vi "MFCCMD.vi"(8 "error in (no error)":errorcluster, 9 "cmd":string, 10 "Device ID's":string[](array[string]), 11 "VISA Refnum in":refnum<visa-resource-name>) -> (0 "error out":errorcluster, 3 "VISA Refnum out":refnum<visa-resource-name>)   [LabVIEW 2020, in "MFC.lvclass"]
uses:
  MFC/MFC.lvclass
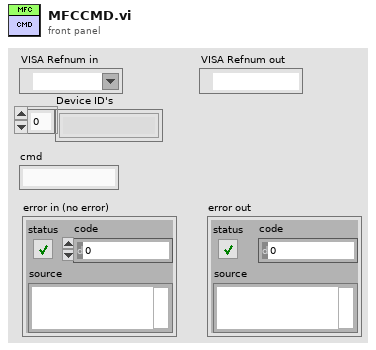
[diagram p1: front panel]
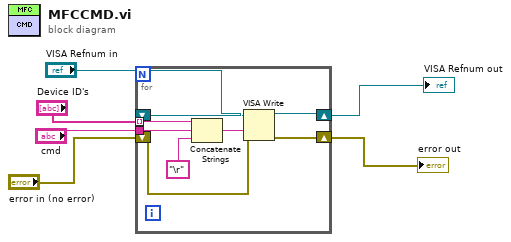
[diagram p0: block diagram]
diagram:
  n1 = for {
    tunnel: "Device ID's" -> [w12] mode=indexing
    shift-right: [w7] -> w5
    shift-left: "error in (no error)" -> [w14]
    shift-right: [w8] -> w6
    shift-left: "VISA Refnum in" -> [w13]
    tunnel: "cmd" -> [w10]
    n2 = Concatenate Strings(w12, w10, "\r" ("string")) -> (w11:string)
    n3 = VISA Write(VISA resource name=w13, write buffer=w11, error in (no error)=w14) -> (VISA resource name out=w8:refnum<visa-resource-name>, error out=w7:errorcluster)  [unwired: 1 out]
  }
  "VISA Refnum out" <- w6
  "error out" <- w5
